vi "LWXPS_PositionerFeedforwardPositionDisable.vi"(6 "LabVIEW error IN":errorcluster, 8 "Positioner Name":string, 9 "XPS Reference IN":refnum<k24>) -> (0 "LabVIEW error OUT":errorcluster, 1 "XPS Error String":string, 2 "Returned error code":i32, 3 "XPS Reference OUT":refnum<k24>)   [LabVIEW 2014]
uses:
  D:/XPSQ8_LabView_Library/Development/Source/Dll/Newport.XPS.CommandInterface.dll
  Dll/Newport.XPS.CommandInterface.dll
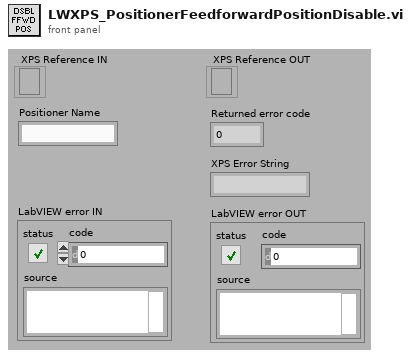
[diagram p1: front panel]
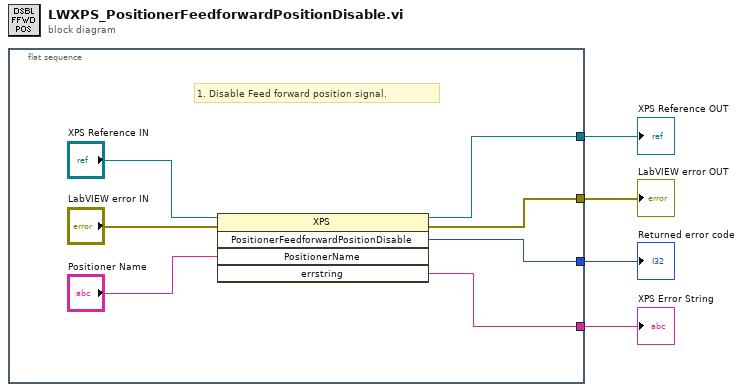
[diagram p0: block diagram]
diagram:
  n1 = flat-sequence {
    tunnel: [w5] -> w1
    tunnel: [w10] -> w4
    tunnel: [w9] -> w3
    tunnel: [w8] -> w2
    frame #0 {
      # "1. Disable Feed forward position signal."
      n2 = invoke class="XPS" method="PositionerFeedforwardPositionDisable"(reference="XPS Reference IN", error in="LabVIEW error IN", "PositionerName"="Positioner Name") -> (reference out=w10:refnum<k24>, error out=w9:errorcluster, "PositionerFeedforwardPositionDisable"=w8:i32, "errstring"=w5:string)  [unwired: 2 in, 1 out]
    }
  }
  "XPS Error String" <- w1
  "XPS Reference OUT" <- w4
  "LabVIEW error OUT" <- w3
  "Returned error code" <- w2
